vi "Problem 67 - Maximum path sum II.vi"() -> ()   [LabVIEW 2021, in "Project Euler.lvlib"]
uses:
  Project Euler.lvlib
panel:
  out "path":string
  out "no. of nodes in path":i32
  out "Answer = maximum total from top to bottom":u64
  out "Triangle of numbers":string="75\n95 64\n17 47 82\n18 35 87 10\n20 04 82 47 65\n19 01 23 75 03 34\n88 02 77 73 07 63 67\n99 65 04 28 06 16 70 92\n41 41 26 56 83 40 80 70 33\n41 48 72 33 47 32 37 16 94 29\n53 71 44 65 25 43 91 52 97 51 14\n70 11 33 28 77 73 17 78 39 68 17 57\n91 71 52 38 17 14 91 43 58 50 27 29 48\n63 66 04 68 89 53 67 30 73 16 69 87 40 31\n04 62 98 27 23 09 70 98 73 93 38 53 60 04 23"
  out "Total execution time (ms)":u32
  # "Input\nInputs to the VI"
  # "Development\nControls or indicators that are useful for development or testing, but which are not outputs of the VI."
  # "Output\nOutputs of the VI"
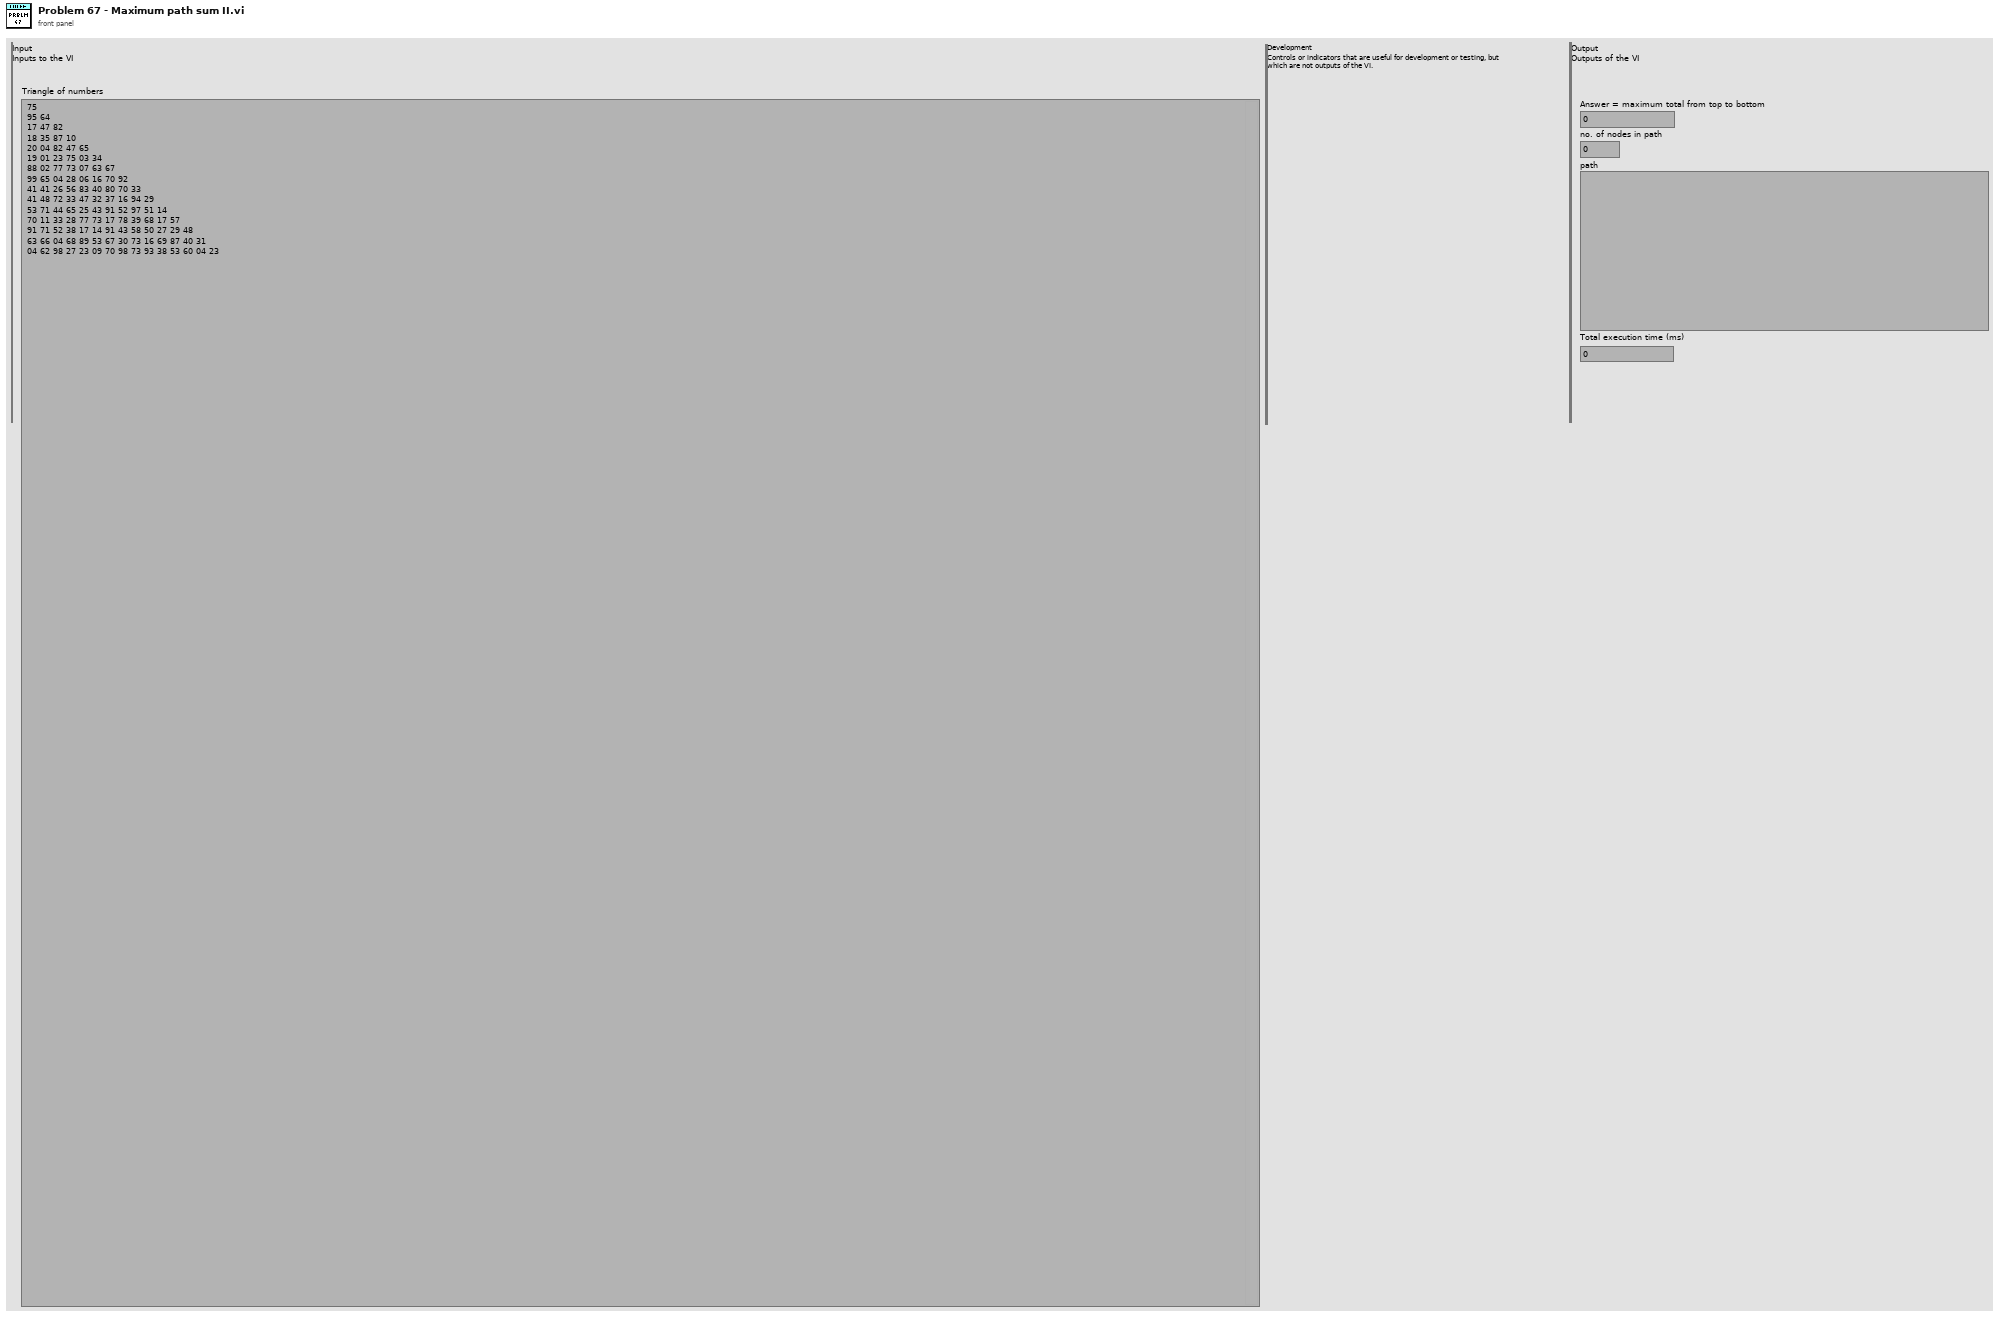
[diagram p1: front panel]
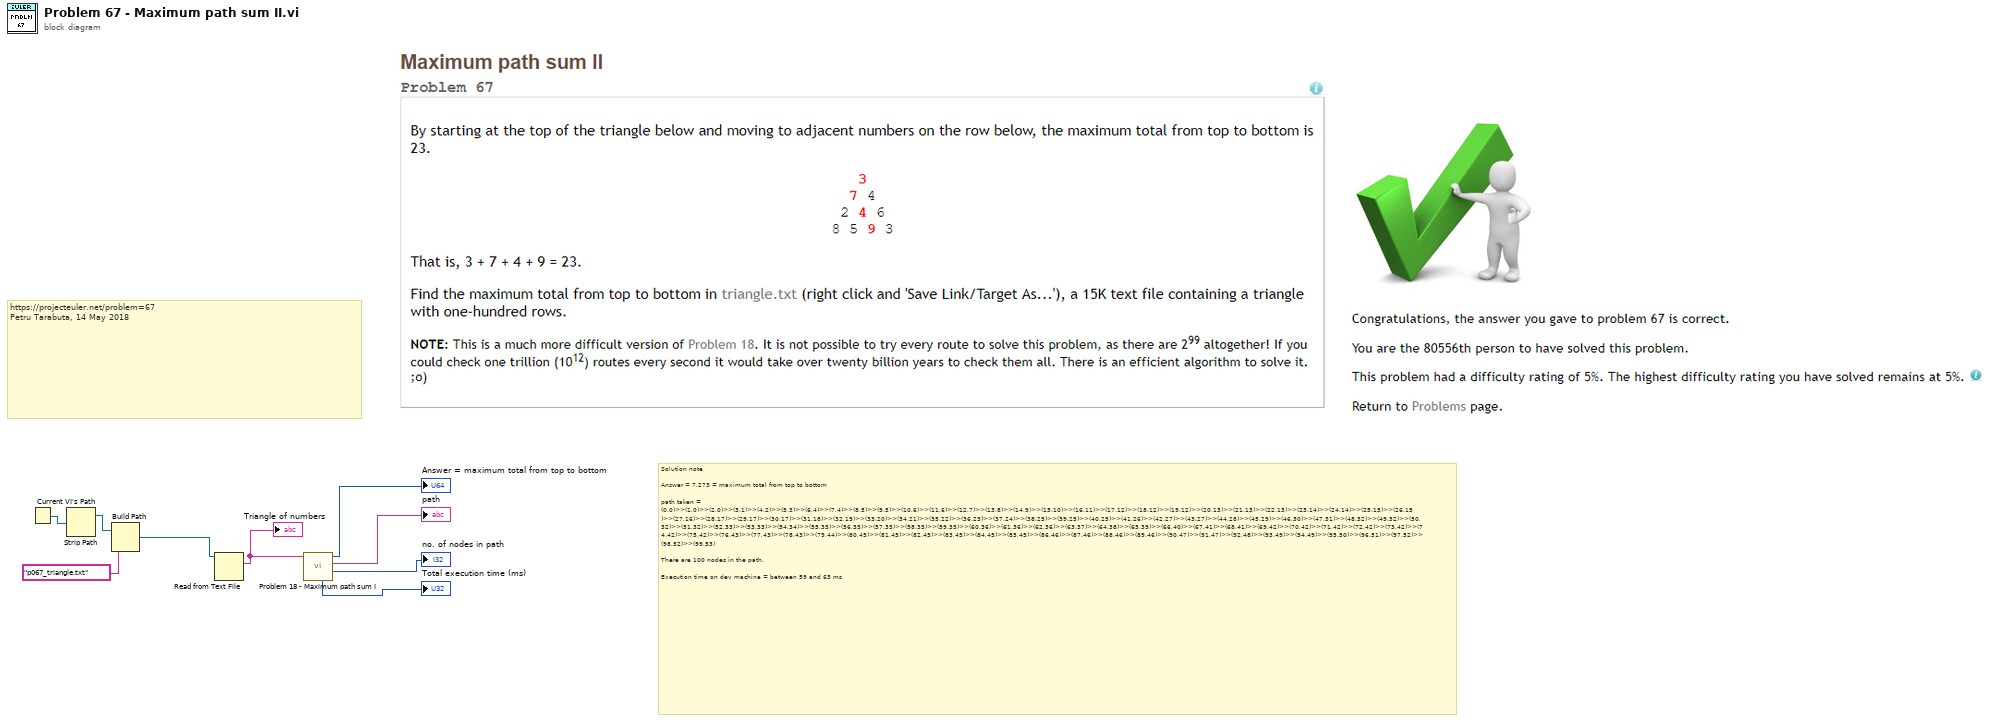
[diagram p0: block diagram]
diagram:
  # "Solution note\n\nAnswer = 7,273 = maximum total from top to bottom\n\npath taken = (0,0)>>(1,0)>>(2,0)>>(3,1)>>(4,2)>>(5,3)>>(6,4)>>(7,4)>>(8,5)>>(9,5)>>(10,6)>>(11,6)>>(12,7)>>(13,8)>>(14,9)>>(15,10)>>(16,11)>>(17,12)>>(18,12)>>(19,12)>>(20,13)>>(21,13)>>(22,13)>>(23,14)>>(24,14)>>(25,15)>>(26,15)>>(27,16)>>(28,17)>>(29,17)>>(30,17)>>(31,18)>>(32,19)>>(33,20)>>(34,21)>>(35,22)>>(36,23)>>(37,24)>>(38,25)>>(39,25)>>(40,25)>>(41,26)>>(42,27)>>(43,27)>>(44,28)>>(45,29)>>(46,30)>>(47,31)>>(48,32)>>(49,32)>>(50,32)>>(51,32)>>(52,33)>>(53,33)>>(54,34)>>(55,35)>>(56,35)>>(57,35)>>(58,35)>>(59,35)>>(60,36)>>(61,36)>>(62,36)>>(63,37)>>(64,38)>>(65,39)>>(66,40)>>(67,41)>>(68,41)>>(69,42)>>(70,42)>>(71,42)>>(72,42)>>(73,42)>>(74,42)>>(75,42)>>(76,43)>>(77,43)>>(78,43)>>(79,44)>>(80,45)>>(81,45)>>(82,45)>>(83,45)>>(84,45)>>(85,45)>>(86,46)>>(87,46)>>(88,46)>>(89,46)>>(90,47)>>(91,47)>>(92,48)>>(93,49)>>(94,49)>>(95,50)>>(96,51)>>(97,52)>>(98,52)>>(99,53)\n\nThere are 100 nodes in the path.\n\nExecution time on dev machine = between 59 and 63 ms"
  # "https://projecteuler.net/problem=67\nPetru Tarabuta, 14 May 2018"
  n1 = Current VI's Path() -> (path=w2:path)
  n2 = Strip Path(path=w2) -> (stripped path=w1:path)  [unwired: 1 out]
  n3 = Build Path(base path=w1, name or relative path="p067_triangle.txt") -> (appended path=w3:path)
  n4 = Read from Text File(file (use dialog)=w3) -> (text=w5:string)  [unwired: 3 in, 3 out]
  "Triangle of numbers" <- w5
  n5 = call "Problem 18 - Maximum path sum I.vi"("Triangle of numbers"=w5) -> ("no. of nodes in path"=→"no. of nodes in path":i32, "path"=→"path":string, "Answer = maximum total from top to bottom"=→"Answer = maximum total from top to bottom":u64, "Total execution time (ms)"=→"Total execution time (ms)":u32)  [unwired: 7 in]
